vi "Gasteiler2String.vi"(11 "Cluster Array (Eingang)":T1[](array[typedef]) {"Gasteiler Letzte Wartung" format="%<%x %.3X>T"}) -> (3 "Gasteiler definition":string[][](array[string]))   [LabVIEW 2020, in "System Einstellungen V2.lvlib"]
uses:
  System Einstellungen V2.lvlib
  Gasteiler.ctl
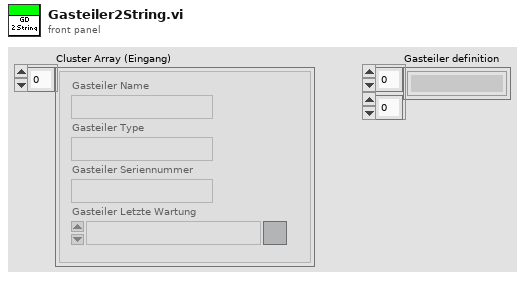
[diagram p1: front panel]
types:
  T1 = typedef "System Einstellungen V2.lvlib/Gasteiler.ctl" = cluster{"Gasteiler Name":string, "Gasteiler Type":string, "Gasteiler Seriennummer":string, "Gasteiler Letzte Wartung":timestamp}
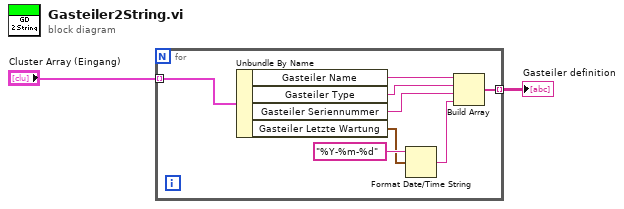
[diagram p0: block diagram]
diagram:
  n1 = for {
    tunnel: "Cluster Array (Eingang)" -> [w10] mode=indexing
    tunnel: [w6] -> w1 mode=indexing
    n2 = Unbundle By Name(w10) -> ("Gasteiler Name"=w9:string, "Gasteiler Type"=w8:string, "Gasteiler Seriennummer"=w7:string, "Gasteiler Letzte Wartung"=w4:timestamp)
    n3 = Format Date/Time String(time format string (%c)="%Y-%m-%d" ("Zeitformatierungs-String (%c)"), seconds (now)=w4) -> (date/time string=w3:string)  [unwired: 1 in]
    n4 = Build Array(w9, w8, w7, w3) -> (w6:string[])
  }
  "Gasteiler definition" <- w1
